vi "Capture@Display2User__Parameter.vi"(1 "ParamterIn":string) -> (0 "ParamterOut":string)   [LabVIEW 2019]
panel:
  in  "RefName":string(combo)
  in  "CamName":string(combo)
  in  "Confirm":bool
  # "Capture@Display2User $Capture,$UserPanelControlName"
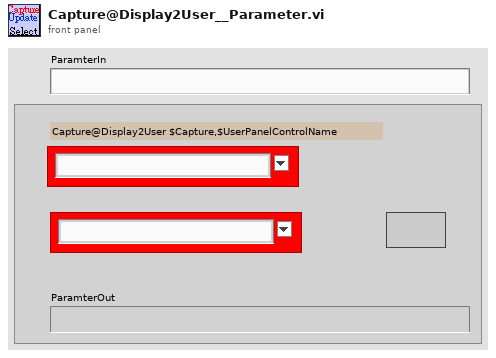
[diagram p1: front panel]
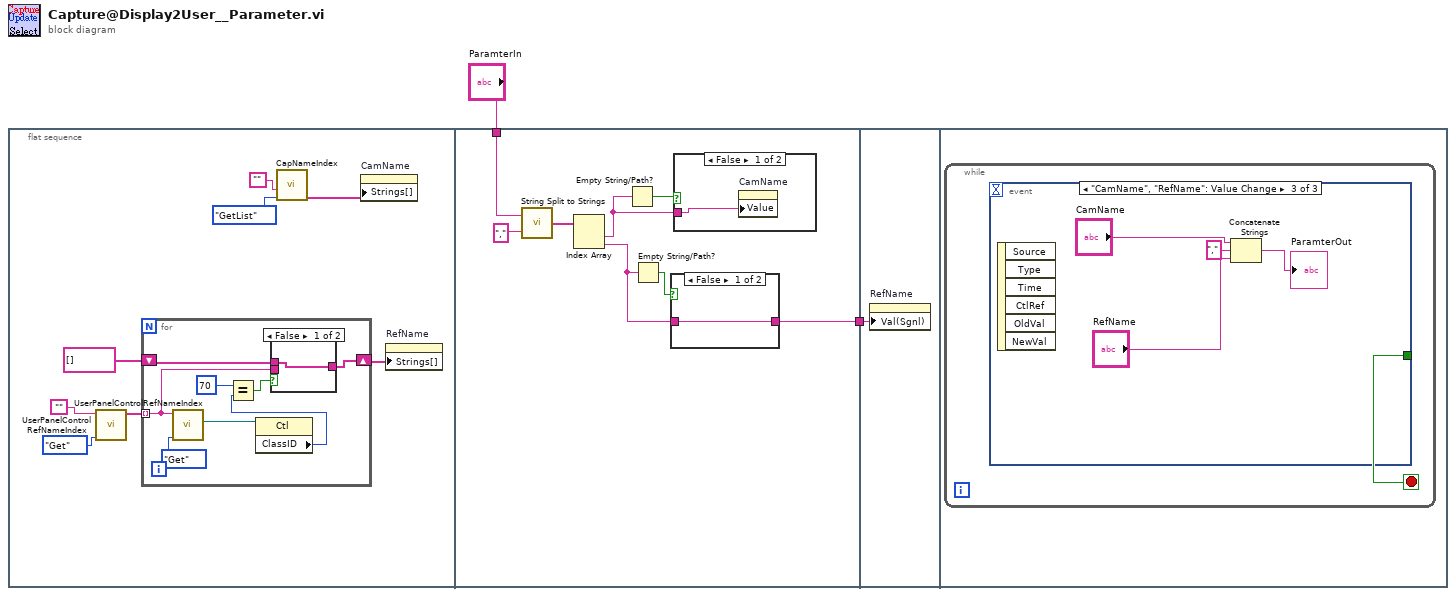
[diagram p0: block diagram]
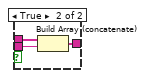
[diagram p2: hidden frame]
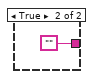
[diagram p3: hidden frame]
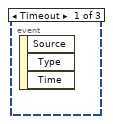
[diagram p5: hidden frame]
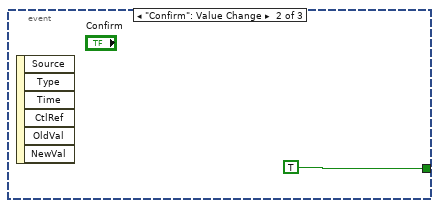
[diagram p6: hidden frame]
diagram:
  n1 = flat-sequence {
    tunnel: "ParamterIn" -> [w26]
    tunnel: [w23] -> w1
    tunnel: w1 -> [w34]
    frame #0 {
      n2 = call "UserPanelControlRefNameIndex.vi"("OP"=enum16{"Get", "Update", "Init"}."Get", "ControlName"="") -> ("ControlNameS"=w7:string[])  [unwired: 6 in, 3 out]
      n3 = for {
        tunnel: w7 -> [w13] mode=indexing
        shift-right: [w12] -> w3
        shift-left: string[] [] ("Strings []") -> [w14]
        n4 = call "UserPanelControlRefNameIndex.vi"("OP"=enum16{"Get", "Update", "Init"}."Get", "ControlName"=w13) -> ("ControlRefOut"=w17:refnum<vi>)  [unwired: 6 in, 3 out]
        n5 = property class="Ctl"(reference=w17) -> ("ClassID"=w16:u32)  [unwired: 1 in, 2 out]
        n6 = Equal?(x=u32 70, y=w16) -> (x = y?=w15:bool)
        n7 = case shown="False" w15 {
          tunnel: w14 -> [w19 w22]
          tunnel: w13 -> [_ w21]
          tunnel: [w19 w20] -> w12
          frame False {
          }
          frame True {
            n8 = Build Array (concatenate)(w22, w21) -> (w20:string[])
          }
        }
      }
      n9 = call "CapNameIndex.vi"("OP"=enum16{"AddCam", "GetIndex", "Init", "GetList"}."GetList", "CamName"="") -> ("DeviceList"=w9:string[])  [unwired: 2 in, 3 out]
      n10 = property on="CamName" class="CmbBox"("Strings[]"=w9) -> ()  [unwired: 2 in, 2 out]
      n11 = property on="RefName" class="CmbBox"("Strings[]"=w3) -> ()  [unwired: 2 in, 2 out]
    }
    frame #1 {
      n12 = call "String Split to Strings.vi"("search string/char (-)"=",", "String"=w26) -> ("Array"=w27:string[])
      n13 = Index Array(array=w27) -> (element #1=w25:string, element #2=w24:string)  [unwired: 2 in]
      n14 = Empty String/Path?(string/path=w25) -> (empty?=w30:bool)
      n15 = Empty String/Path?(string/path=w24) -> (empty?=w29:bool)
      n16 = case shown="False" w29 {
        tunnel: [w31 ""] -> w23
        tunnel: w24 -> [w31 _]
        frame False {
        }
        frame True {
        }
      }
      n17 = case shown="False" w30 {
        tunnel: w25 -> [w33 _]
        frame False {
          n18 = property on="CamName" class="CmbBox"("Value"=w33) -> ()  [unwired: 2 in, 2 out]
        }
        frame True {
        }
      }
    }
    frame #2 {
      n19 = property on="RefName" class="CmbBox"("Val(Sgnl)"=w34) -> ()  [unwired: 2 in, 2 out]
    }
    frame #3 {
      n20 = while {
        stop <- w35 stop-if-true
        n21 = event shown="[2] \"CamName\", \"RefName\": Value Change" {
          selector: _ -> [_ _ _]
          dyn-events: _ -> [_ _ _]
          timeout: _ -> [_ _ _]
          tunnel: [_ TRUE _] -> w35
          event Timeout {
            n22 = event-data() -> ()  [unwired: 1 in, 3 out]
          }
          event "Confirm": Value Change {
            n23 = event-data() -> ()  [unwired: 1 in, 6 out]
          }
          event "CamName", "RefName": Value Change {
            n24 = event-data() -> ()  [unwired: 1 in, 6 out]
            n25 = Concatenate Strings("CamName", "," ("string"), "RefName") -> (→"ParamterOut":string)
          }
        }
      }
    }
  }
